vi "VIE.Module.Queued Message Handler.[enqueue].State.PolyChild.QueuedMessageHandler.vi"(6 "Where to Enque (End of the Queue)":enum16{"Start of the Queue", "End of the Queue"}(ring)=enum."End of the Queue", 8 "error in (no error)":errorcluster, 9 "States to Enqueue":string[](array[string]), 10 "QueuedMessageHandler.dqGOOPClass (in)":T1) -> (0 "error out":errorcluster, 2 "QueuedMessageHandler.dqGOOPClass (out)":T1)   [LabVIEW 2010, in "VIE.Module.Queued Message Handler.QueuedMessageHandler.dqGOOPClass.lvlib"]
uses:
  VIE.Module.Queued Message Handler.QueuedMessageHandler.dqGOOPClass.lvlib
  VIE.Module.Queued Message Handler.dqClass_ObjectReference.ctl
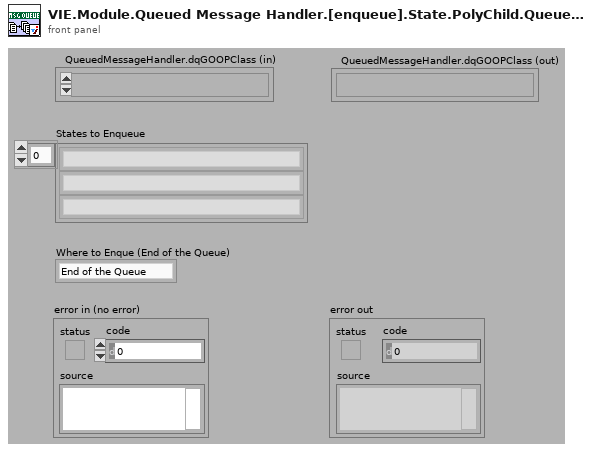
[diagram p1: front panel]
types:
  T1 = typedef "VIE.Module.Queued Message Handler.QueuedMessageHandler.dqGOOPClass.lvlib/VIE.Module.Queued Message Handler.dqClass_ObjectReference.ctl" = refnum<k1>
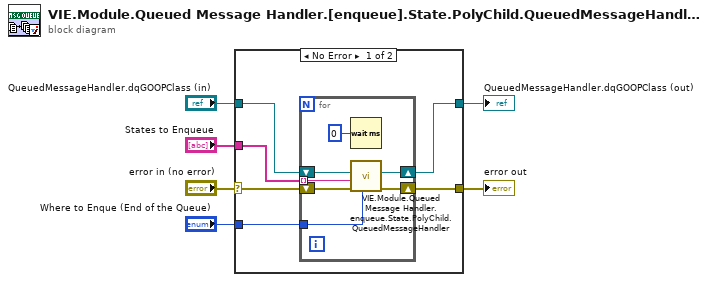
[diagram p0: block diagram]
diagram:
  n1 = case shown="No Error" "error in (no error)" {
    selector: "error in (no error)" -> [w9 w21]
    tunnel: [w10 w21] -> w5
    tunnel: [w11 w20] -> w4
    tunnel: "QueuedMessageHandler.dqGOOPClass (in)" -> [w12 w20]
    tunnel: "States to Enqueue" -> [w8 _]
    tunnel: "Where to Enque (End of the Queue)" -> [w7 _]
    frame No Error {
      n2 = for {
        shift-right: [w16] -> w10
        shift-left: w9 -> [w18]
        tunnel: w8 -> [w17] mode=indexing
        shift-right: [w14] -> w11
        shift-left: w12 -> [w15]
        tunnel: w7 -> [w13]
        n3 = Wait (ms)(milliseconds to wait=u32 0) -> ()  [unwired: 1 out]
        n4 = call "VIE.Module.Queued Message Handler.enqueue.State.PolyChild.QueuedMessageHandler.vi"("Where to Enque (End of the Queue)"=w13, "error in (no error)"=w18, "State to Enqueue"=w17, "QueuedMessageHandler.dqGOOPClass (in)"=w15) -> ("error out"=w16:errorcluster, "QueuedMessageHandler.dqGOOPClass (out)"=w14:T1)  [unwired: 6 in]
      }
    }
    frame Error {
    }
  }
  "error out" <- w5
  "QueuedMessageHandler.dqGOOPClass (out)" <- w4
